vi "GetPulWidth.vi"(8 "错误输入（无错误）":errorcluster) -> (0 "错误输出":errorcluster, 3 "返回值":u32)   [LabVIEW 2018]
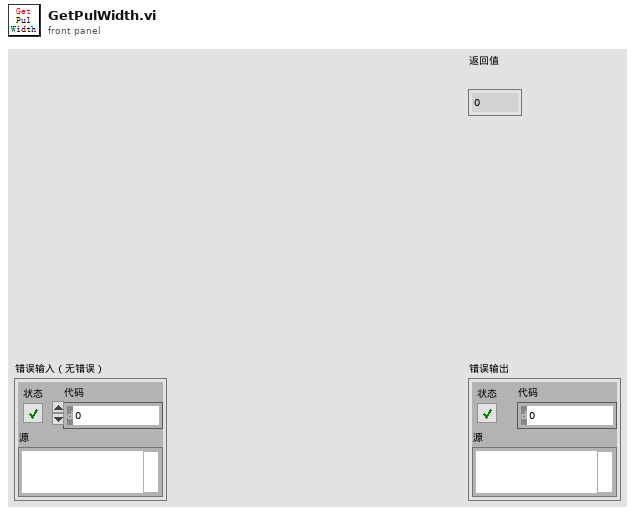
[diagram p1: front panel]
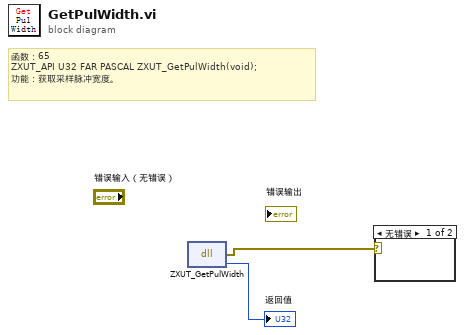
[diagram p0: block diagram]
diagram:
  # "函数：65\nZXUT_API U32\tFAR PASCAL ZXUT_GetPulWidth(void);\n功能：获取采样脉冲宽度。"
  n1 = dll-call lib="PTH2Rabs E软件项目超声超声子VI函数VI\tTCG处理ZXUTConfigMgr.dll" fn="ZXUT_GetPulWidth"() -> (error out=w1:errorcluster, "返回值"=→"返回值":u32)  [unwired: 3 in, 1 out]
  n2 = case shown="无错误" w1 {
    frame No Error {
    }
    frame Error {
    }
  }
